vi "get_nearest.vi"(5 "interval_sec":dbl, 6 "current time":timestamp caption="тв") -> (0 "found":bool, 1 "next_TimeStamp":timestamp, 2 "seconds_remind":dbl)   [LabVIEW 2010]
uses:
  lib/Global 2.vi
panel:
  in  "OK Button":bool caption="Перечитать"
  out "In Range?":bool
  out "Array":timestamp[](array[timestamp]) caption="Расписание" format="%<%X>T"
  # "Найти время в расписании\nв интервале \nот текущего времени (тв)\nдо тв+interval_sec."
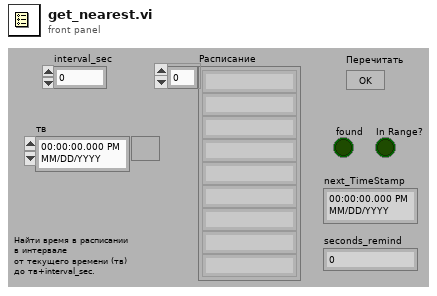
[diagram p1: front panel]
types:
  T1 = typedef "LVDateTimeRec.ctl" = cluster{"fractional second":dbl, "second":i32, "minute":i32, "hour":i32, "day of month":i32, "month":i32, "year":i32, "day of week":i32, "day of year":i32, "DST":i32}
  T2 = enum16{"read/write", "read-only", "write-only", "write-only (truncate)"}
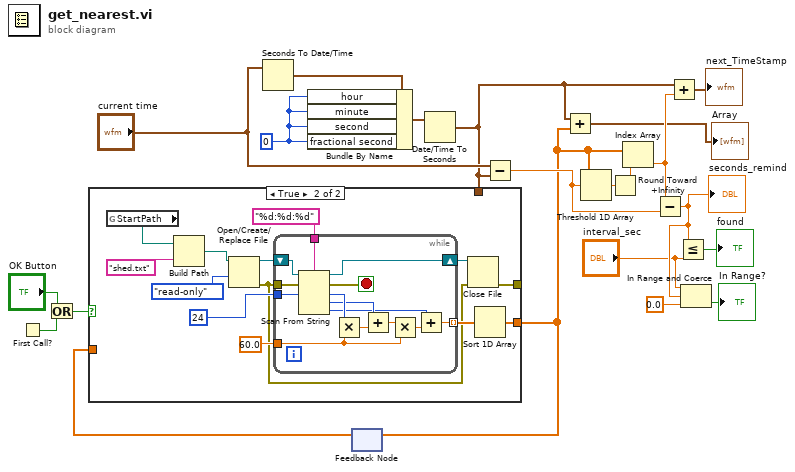
[diagram p0: block diagram]
diagram:
  w20 = 0 ("hour")
  n1 = First Call?() -> (First Call?: T/F=w2:bool)
  n2 = Or(x="OK Button", y=w2) -> (x .or. y?=w1:bool)
  n3 = Seconds To Date/Time(time stamp (now)="current time") -> (date time rec=w21:T1)  [unwired: 1 in]
  n4 = Bundle By Name(cluster=w21, "hour"=w20, "minute"=w20, "second"=w20, "fractional second"=w20) -> (w17:T1)
  n5 = feedback #1() -> (w11:dbl[])  [unwired: 1 in]
  n6 = Date/Time To Seconds(2:w17) -> (0:w5:timestamp)  [unwired: 1 in]
  n7 = case shown="True" w1 {
    tunnel: [w22 w28] -> w6
    tunnel: w11 -> [w22 _]
    tunnel: w5 -> [_ _]
    tunnel: [_ w23] -> _
    frame False {
    }
    frame True {
      n8 = global read "Global 2.vi" "StartPath"() -> (w25:path)
      n9 = Build Path(base path=w25, name or relative path="shed.txt") -> (appended path=w33:path)
      n10 = Open/Create/Replace File(file path (use dialog)=w33, access (0:read/write)=T2."read-only" ("open mode (0)")) -> (refnum out=w34:refnum<file>, error out=w24:errorcluster)  [unwired: 4 in, 1 out]
      n11 = while {
        tunnel: "%d:%d:%d" ("format string") -> [w49]
        shift-right: [w47] -> w32
        shift-left: w34 -> [w48]
        tunnel: 60.0 -> [w40]
        tunnel: [w37] -> w26 mode=indexing
        tunnel: w24 -> [w46]
        tunnel: 24 -> [w36]
        stop <- w45 stop-if-true
        n12 = Scan From String(w49, w48, w46, default 1=w36) -> (w47:refnum<file>, w45:errorcluster, output 1=w44:i32, output 2=w42:i32, output 3=w38:i32)  [unwired: 2 in]
        n13 = Multiply(x=w44, y=w40) -> (x*y=w43:dbl)
        n14 = Add(x=w42, y=w43) -> (x+y=w41:dbl)
        n15 = Multiply(x=w41, y=w40) -> (x*y=w39:dbl)
        n16 = Add(x=w38, y=w39) -> (x+y=w37:dbl)
      }
      n17 = Close File(refnum=w32, error in=w24) -> (error out=w23:errorcluster)  [unwired: 1 out]
      n18 = Sort 1D Array(array=w26) -> (sorted array=w28:dbl[])
    }
  }
  n19 = feedback-in #1(w6) -> ()
  n20 = Subtract(x="current time", y=w5) -> (x-y=w15:dbl)
  n21 = Add(x=w5, y=w6) -> (x+y=→"Array":timestamp[])
  n22 = Threshold 1D Array(2:w15, 3:w6) -> (0:w19:dbl)  [unwired: 1 in]
  n23 = Round Toward +Infinity(x=w19) -> (ceil(x): smallest int >= x=w18:dbl)
  n24 = Index Array(array=w6, index=w18) -> (element=w14:dbl)
  n25 = Subtract(x=w14, y=w15) -> (x-y=w10:dbl)
  "seconds_remind" <- w10
  n26 = Add(x=w5, y=w14) -> (x+y=→"next_TimeStamp":timestamp)
  n27 = Less Or Equal?(x=w10, y="interval_sec") -> (x <= y?=→"found":bool)
  n28 = In Range and Coerce(upper limit="interval_sec", x=w10, lower limit=0.0) -> (In Range?=→"In Range?":bool)  [unwired: 1 out]
